vi "LED Example.vi"() -> ()   [LabVIEW 2016]
panel:
  in  "LED Strip Pin":T1(ring)=enum."HB GPIO 0"
  in  "Strip Length":u8=100
  in  "LED Model":enum8{"WS2812", "WS2812B"}(ring)
  in  "LED Color":u32(colorbox)=786687
  in  "stop":bool
  in  "Update Frequency":dbl(slide)=2.428365068313236 scale=0.1..20.0
  # "Set these controls before running the example"
  # "This example demonstrates how to write data to a file on the SD card of the Huskie Board.\n\nSpecify the file name and the header string before running the example. The file name must conform to \"8.3' file name conventions. That is there can be at most eight characters followed by a period followed by a three character extension.\n\nThe reminaing controls may be changed while the example is running. All values written to the log must be strings. This example shows how to convert numbers to strings before invoking the HB_WriteToLog VI.\n\nPlease note that only one file may be open at a time."
  # "Change these controls while running the example"
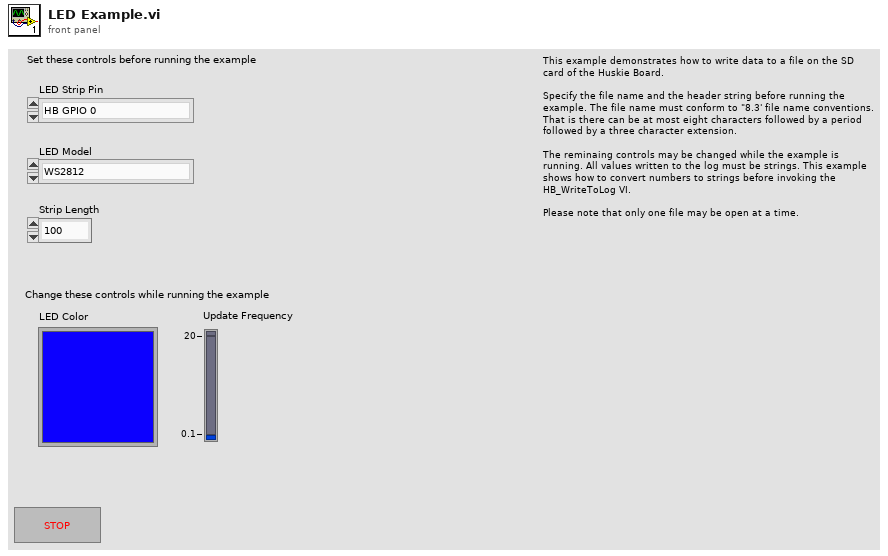
[diagram p1: front panel]
types:
  T1 = enum8{"SD card D1", "SD card D0", "SD card CLK", "SD card CMD", "SD card D2", "SD card D3", "roboRIO MOSI", "roboRIO MISO", "roboRIO CLK", "roboRIO CS", "roboRIO UART RX", "roboRIO UART TX", "roboRIO SCL", "robotRIO SDA", "HB GPIO 0", "HB GPIO 1", "HB GPIO 2", "HB GPIO 3", "HB LCD", "ADC CS2", "ADC CS1", "ADC DO", "ADC CLK", "ADC DI", "LED 1", "LED 2", "LED 3", "LED 4", "EEPROM SCL", "EEPROM SDA", "USB UART TX", "USB UART RX"}
  T2 = typedef "WPI_SerialPortRef.ctl" = cluster{"DevStatus":errorcluster, "Serial Port Name":refnum<visa-resource-name>}
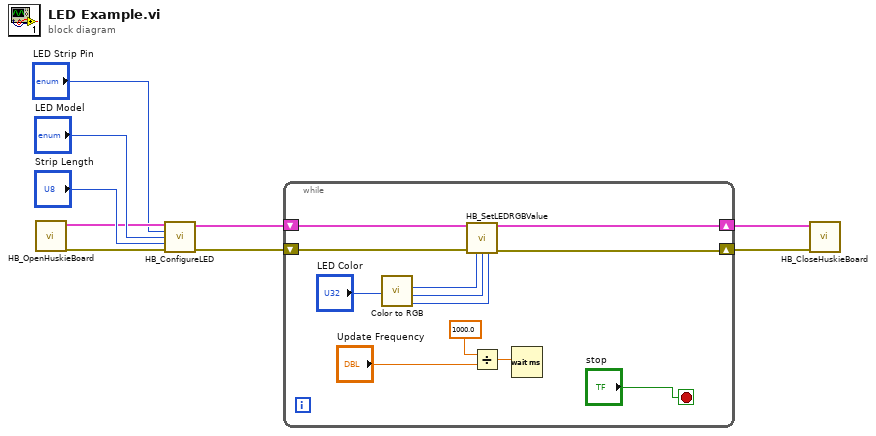
[diagram p0: block diagram]
diagram:
  n1 = call <vilib>:"HB_OpenHuskieBoard.vi"() -> ("error out"=w5:errorcluster, "HBDeviceRef"=w2:T2)  [unwired: 10 in]
  n2 = call <vilib>:"HB_ConfigureLED.vi"("HBDevRef"=w2, "LED Strip Pin"="LED Strip Pin", "LED Model"="LED Model", "Number of LEDs"="Strip Length", "error in (no error)"=w5) -> ("HBDevRef"=w7:T2, "error out"=w6:errorcluster)  [unwired: 9 in]
  n3 = while {
    shift-right: [w14] -> w8
    shift-left: w7 -> [w17]
    shift-right: [w15] -> w9
    shift-left: w6 -> [w16]
    stop <- "stop" stop-if-true
    n4 = call <vilib>:"Color to RGB.vi"("Color"="LED Color") -> ("R"=w12:u8, "G"=w11:u8, "B"=w10:u8)  [unwired: 1 out]
    n5 = call <vilib>:"HB_SetLEDRGBValue.vi"("HBDevRef"=w17, "error in (no error)"=w16, "Red"=w12, "Green"=w11, "Blue"=w10) -> ("HBDevRef"=w14:T2, "error out"=w15:errorcluster)  [unwired: 9 in]
    n6 = Divide(x=1000.0, y="Update Frequency") -> (x/y=w20:dbl)
    n7 = Wait (ms)(milliseconds to wait=w20) -> ()  [unwired: 1 out]
  }
  n8 = call <vilib>:"HB_CloseHuskieBoard.vi"("error in (no error)"=w9, "HBDeviceRef"=w8) -> ()  [unwired: 9 in, 1 out]
